vi "Variant to String.vi"(8 "error in (no error)":errorcluster, 11 "Data (Variant)":variant) -> (0 "error out":errorcluster, 3 "String":string)   [LabVIEW 2019, in "LV-Data.lvclass"]
uses:
  LV-Data.lvclass
  <vilib>/Utility/error.llb/Error Cluster From Error Code.vi
  <vilib>/ErrorRing/Error Ring.xnode
  <vilib>/Utility/Data Type/NI_Data Type.lvlib
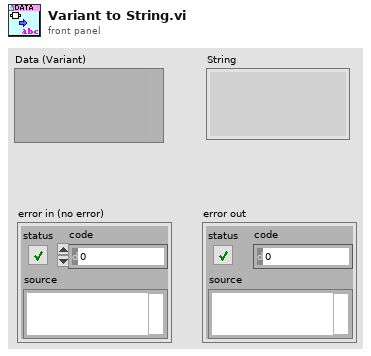
[diagram p1: front panel]
types:
  T1 = typedef "NI_Data Type.lvlib/Data Type.ctl" = enum8{"Invalid Type", "Void", "I8", "I16", "I32", "I64", "U8", "U16", "U32", "U64", "Single Float", "Double Float", "Extended Float", "Single Complex", "Double Complex", "Extended Complex", "Enum U8", "Enum U16", "Enum U32", "Enum U64", "Single Float With Unit", "Double Float With Unit", "Extended Float With Unit", "Single Complex with Unit", "Double Complex with Unit", "Extended Complex with Unit", "Boolean", "String", "Path", "Picture", "Tag", "Array", "Cluster", "Variant", "LV Variant", "Waveform", "Timestamp", "Digital Waveform", "Digital Data", "ExpressData", "Refnum", "External Data", "VI", "Poly VI", "LabVIEW Class Instance", "Fixed Point", "Set Collection", "Map Collection"}
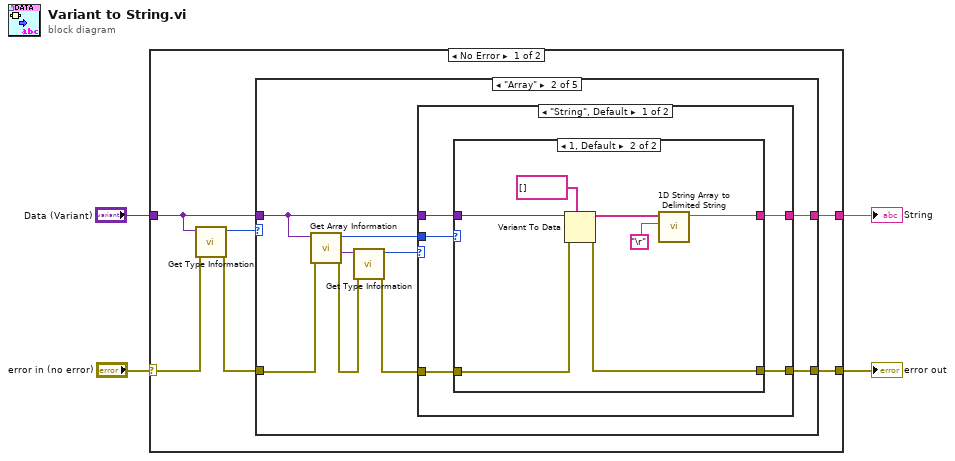
[diagram p0: block diagram]
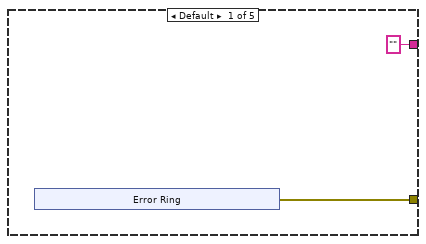
[diagram p2: hidden frame]
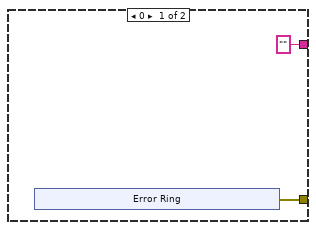
[diagram p3: hidden frame]
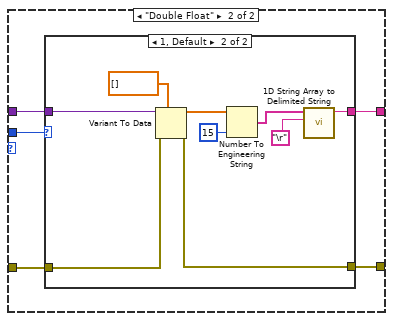
[diagram p4: hidden frame]
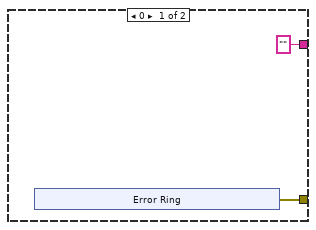
[diagram p5: hidden frame]
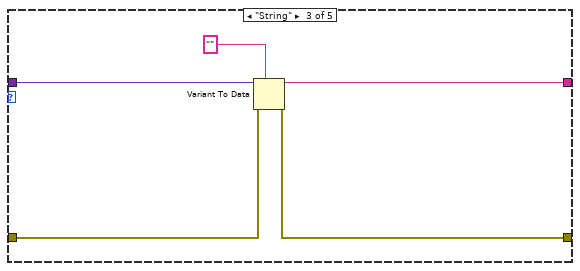
[diagram p6: hidden frame]
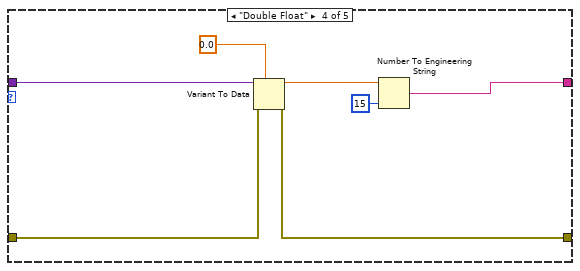
[diagram p7: hidden frame]
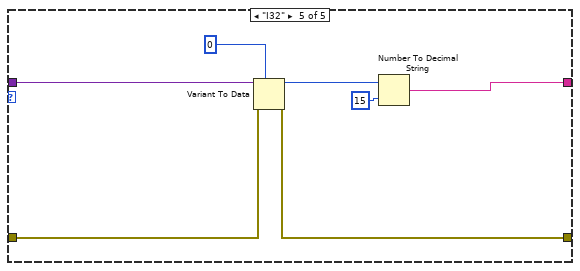
[diagram p8: hidden frame]
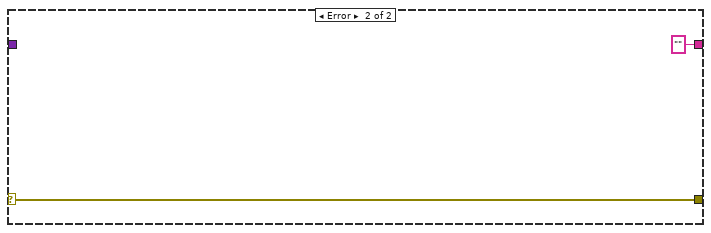
[diagram p9: hidden frame]
diagram:
  n1 = case shown="No Error" "error in (no error)" {
    selector: "error in (no error)" -> [w7 w84]
    tunnel: [w8 w84] -> w4
    tunnel: "Data (Variant)" -> [w5 _]
    tunnel: [w6 "" ("delimited string")] -> w1
    frame No Error {
      n2 = call <vilib>:"Get Type Information.vi"("error in (no error)"=w7, "variant"=w5) -> ("error out"=w9:errorcluster, "type"=w10:T1)  [unwired: 5 in, 3 out]
      n3 = case shown="\"Array\"" w10 {
        tunnel: [w12 w25 w66 w73 w80] -> w8
        tunnel: w5 -> [_ w24 w68 w75 w82]
        tunnel: w9 -> [_ w23 w67 w74 w81]
        tunnel: ["" ("delimited string") w17 w64 w69 w76] -> w6
        frame Default {
          n4 = xnode "Error Ring"() -> ("error out"=w12:errorcluster)
        }
        frame "Array" {
          n5 = call <vilib>:"Get Array Information.vi"("error in (no error)"=w23, "variant"=w24) -> ("error out"=w21:errorcluster, "array element data type"=w22:variant, "number of dimensions"=w18:i32)  [unwired: 6 in, 1 out]
          n6 = call <vilib>:"Get Type Information.vi"("error in (no error)"=w21, "variant"=w22) -> ("error out"=w20:errorcluster, "type"=w19:T1)  [unwired: 5 in, 3 out]
          n7 = case shown="\"String\", Default" w19 {
            tunnel: [w30 w48] -> w25
            tunnel: w24 -> [w29 w47]
            tunnel: w20 -> [w28 w46]
            tunnel: w18 -> [w27 w45]
            tunnel: [w26 w44] -> w17
            frame "String", Default {
              n8 = case shown="1, Default" w27 {
                tunnel: [w32 w40] -> w30
                tunnel: w29 -> [_ w42]
                tunnel: w28 -> [_ w41]
                tunnel: ["" ("delimited string") w37] -> w26
                frame 0 {
                  n9 = xnode "Error Ring"() -> ("error out"=w32:errorcluster)
                }
                frame 1, Default {
                  n10 = Variant To Data(error in=w41, type=string[] [], Variant=w42) -> (data=w39:string[], error out=w40:errorcluster)
                  n11 = call <vilib>:"1D String Array to Delimited String.vi"("delimiter"="\r", "string array"=w39) -> ("delimited string"=w37:string)  [unwired: 9 in]
                }
              }
            }
            frame "Double Float" {
              n12 = case shown="1, Default" w45 {
                tunnel: [w50 w60] -> w48
                tunnel: w47 -> [_ w62]
                tunnel: w46 -> [_ w61]
                tunnel: ["" ("delimited string") w56] -> w44
                frame 0 {
                  n13 = xnode "Error Ring"() -> ("error out"=w50:errorcluster)
                }
                frame 1, Default {
                  n14 = Variant To Data(error in=w61, type=dbl[] [], Variant=w62) -> (data=w58:dbl[], error out=w60:errorcluster)
                  n15 = Number To Engineering String(2:i16 15 ("precision (6)"), 4:w58) -> (0:w55:string[])  [unwired: 2 out]
                  n16 = call <vilib>:"1D String Array to Delimited String.vi"("delimiter"="\r", "string array"=w55) -> ("delimited string"=w56:string)  [unwired: 9 in]
                }
              }
            }
          }
        }
        frame "String" {
          n17 = Variant To Data(error in=w67, type="", Variant=w68) -> (data=w64:string, error out=w66:errorcluster)
        }
        frame "Double Float" {
          n18 = Variant To Data(error in=w74, type=0.0, Variant=w75) -> (data=w70:dbl, error out=w73:errorcluster)
          n19 = Number To Engineering String(2:i16 15 ("precision (6)"), 4:w70) -> (0:w69:string)  [unwired: 2 out]
        }
        frame "I32" {
          n20 = Variant To Data(error in=w81, type=0, Variant=w82) -> (data=w77:i32, error out=w80:errorcluster)
          n21 = Number To Decimal String(number=w77, width (-)=i16 15 ("precision (6)")) -> (decimal integer string=w76:string)
        }
      }
    }
    frame Error {
    }
  }
  "String" <- w1
  "error out" <- w4
